vi "DATA in.vi"(6 "출력 클러스터":T1, 7 "Retrieved Data.lvclass":refnum<class "Retrieved Data.lvclass">) -> (3 "Retrieved Data.lvclass 2":refnum<class "Retrieved Data.lvclass">)   [LabVIEW 2017, in "Retrieved Data.lvclass"]
uses:
  Retrieved Data.lvclass
  Retrieved Data.lvclass/Retrieved Data.ctl
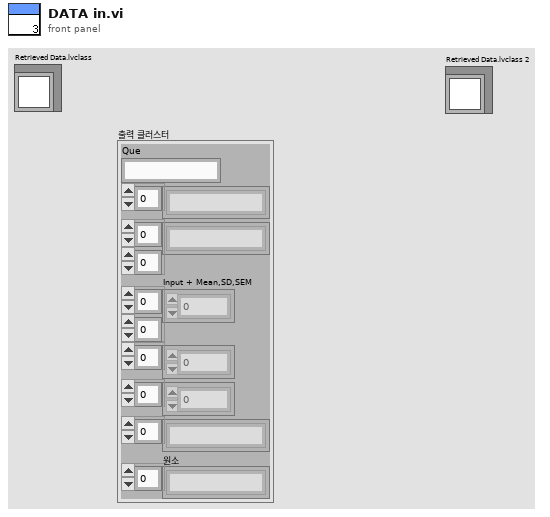
[diagram p1: front panel]
types:
  T1 = cluster{"Que":string, string[], string[][], "Input + Mean,SD,SEM":dbl[][], dbl[], dbl[], string[], "원소":string[]}
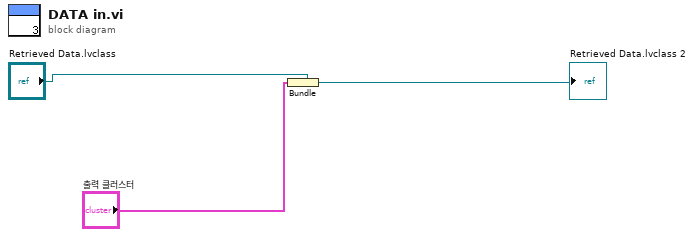
[diagram p0: block diagram]
diagram:
  n1 = Bundle(cluster="Retrieved Data.lvclass", "출력 클러스터") -> (→"Retrieved Data.lvclass 2":refnum<class "Retrieved Data.lvclass">)
